vi "list_sub_tables.vi"(8 "error in (no error)":errorcluster, 11 "Table in":refnum<class "Table.lvclass">) -> (0 "error out":errorcluster, 2 "sub_tables":string[](array[string]), 3 "Table out":refnum<class "Table.lvclass">)   [LabVIEW 2020]
uses:
  toml_edit.lvlib
  dragon_toml_64.dll
  Table.lvclass
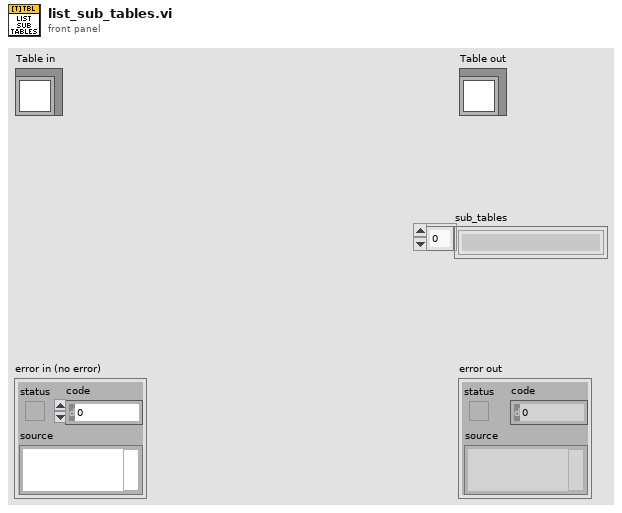
[diagram p1: front panel]
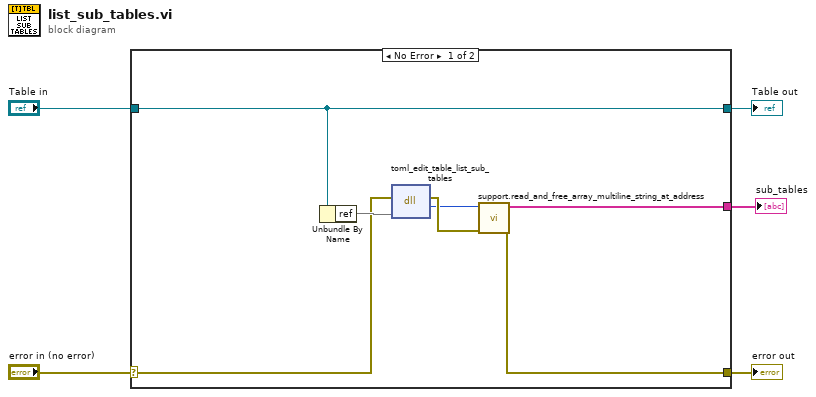
[diagram p0: block diagram]
diagram:
  n1 = case shown="No Error" "error in (no error)" {
    selector: "error in (no error)" -> [w8 w14]
    tunnel: [w7 w14] -> w4
    tunnel: [w9 w13] -> w2
    tunnel: "Table in" -> [w9 w13]
    tunnel: [w6 _] -> w1
    frame No Error {
      n2 = Unbundle By Name(w9) -> ("ref"=w10)
      n3 = dll-call lib="C:/Projects/toml-edit-labview/lv_src/dragon_toml_*.dll" fn="toml_edit_table_list_sub_tables"(error in=w8, "table_ref"=w10) -> (error out=w12:errorcluster, "sub_table_names_ptr"=w11:u64)  [unwired: 3 in, 1 out]
      n4 = call "support.read_and_free_array_multiline_string_at_address.vi"("error in (no error)"=w12, "table_names_ptr"=w11) -> ("error out"=w7:errorcluster, "lines"=w6:string[])  [unwired: 8 in]
    }
    frame Error {
    }
  }
  "error out" <- w4
  "Table out" <- w2
  "sub_tables" <- w1
